vi "Write_parameter.vi"(8 "error in (no error)":errorcluster caption="entrée d'erreur (pas d'erreur)", 10 "Parameter":string, 11 "Class Instrument Multimeter en entrée":refnum<class "Class Instrument LED_Analyser.lvclass">) -> (0 "error out":errorcluster caption="sortie d'erreur", 3 "Class Instrument Multimeter en sortie":refnum<class "Class Instrument LED_Analyser.lvclass">)   [LabVIEW 2020, in "Library Instrument & Equipement.lvlib" / "Library Instruments.lvlib" / "Class Instrument LED_Analyser.lvclass"]
uses:
  Class Instrument LED_Analyser.lvclass
  Commun VI/TypeDef/Commande Led_Analyser/Parametre LED analyser.ctl
  LED Analyser/Class Led Analyser (Default)/Class LED Analyser (Default).lvclass
  JSON API/JSON Value/Set from JSON string.vi
  Instrument (Default)/Class Instrument (Default).lvclass
  JSON API/JSON Value/JSON Value.lvclass
  Class Instrument LED_Analyser.lvclass/Class Instrument LED_Analyser.ctl
  JSON API/Variant JSON/Variant JSON.lvlib
  JSON API/Get Polymorphic/JSON GetSet.lvlib
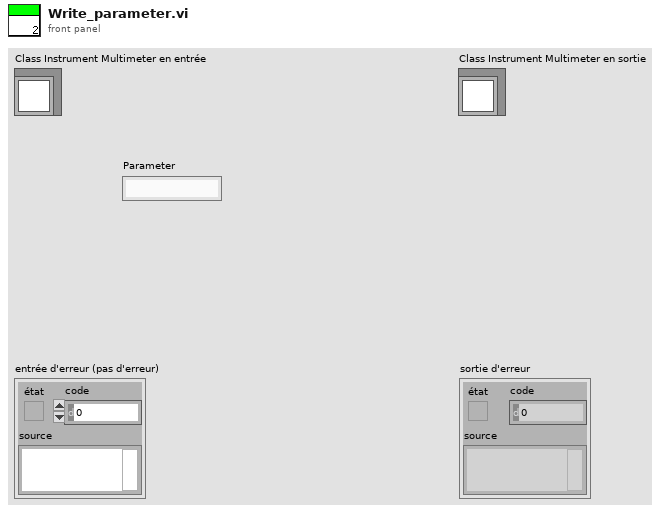
[diagram p1: front panel]
types:
  T1 = typedef "Parametre LED analyser.ctl" = cluster{"Device @":string, "Channel":u16, "LED Analyser":refnum<class "Class LED Analyser (Default).lvclass">}
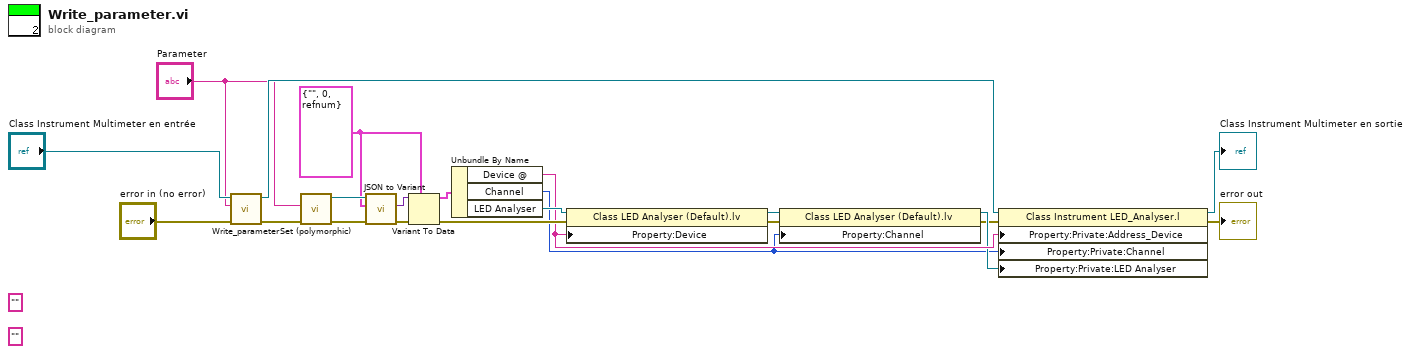
[diagram p0: block diagram]
diagram:
  (unwired) "" ("Device")
  (unwired) "" ("Device")
  w9 = T1 {"Device @"="", "Channel"=0, "LED Analyser"=refnum} ("Parameter")
  n1 = call-parent "Write_parameter.vi"("error in (no error)"="error in (no error)", "Parameter"="Parameter", "Class Instrument (Default) en entrée"="Class Instrument Multimeter en entrée") -> ("error out"=w13:errorcluster, "Class Instrument (Default) en sortie"=w12:refnum<class "Class Instrument LED_Analyser.lvclass">)  [unwired: 7 in]
  n2 = call-poly "Set (polymorphic).vi"("error in (no error)"=w13, "JSON stream"="Parameter") -> ("error out"=w19:errorcluster, "JSON Value out"=w21:refnum<class "JSON Value.lvclass">)  [unwired: 7 in, 1 out]
  n3 = call "JSON to Variant.vi"("error in (no error)"=w19, "Variant (Data Type)"=w9, "JSON Value"=w21) -> ("error out"=w20:errorcluster, "Variant out"=w18:variant)  [unwired: 7 in]
  n4 = Variant To Data(error in=w20, type=w9, Variant=w18) -> (data=w15:T1, error out=w6:errorcluster)
  n5 = Unbundle By Name(w15) -> ("Device @"=w5:string, "Channel"=w3:u16, "LED Analyser"=w8:refnum<class "Class LED Analyser (Default).lvclass">)
  n6 = property class="Class LED Analyser (Default).lv"(reference=w8, error in=w6, "Property:Device"=w5) -> (reference out=w7:refnum<class "Class LED Analyser (Default).lvclass">, error out=w1:errorcluster)
  n7 = property class="Class LED Analyser (Default).lv"(reference=w7, error in=w1, "Property:Channel"=w3) -> (reference out=w4:refnum<class "Class LED Analyser (Default).lvclass">, error out=w2:errorcluster)
  n8 = property class="Class Instrument LED_Analyser.l"(reference=w12, error in=w2, "Property:Private:Address_Device"=w5, "Property:Private:Channel"=w3, "Property:Private:LED Analyser"=w4) -> (reference out=→"Class Instrument Multimeter en sortie":refnum<class "Class Instrument LED_Analyser.lvclass">, error out=→"error out":errorcluster)
